vi "json Delete - string path.vi"(8 "error in (no error)":errorcluster, 10 "path":string, 11 "JSON Document in":refnum<class "JSON Document.lvclass">) -> (0 "error out":errorcluster, 1 "found?":bool, 3 "JSON Document out":refnum<class "JSON Document.lvclass">)   [LabVIEW 2015, in "JSON Document.lvclass"]
uses:
  JSON Document.lvclass
  JSON Document.lvclass/JSON Document.ctl
  rapidjson wrapper/rapidjson wrapper.lvlib
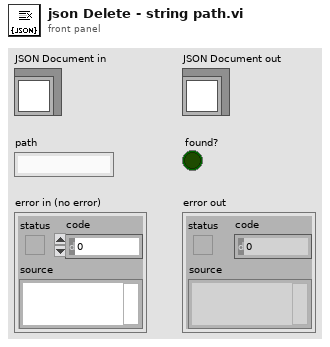
[diagram p1: front panel]
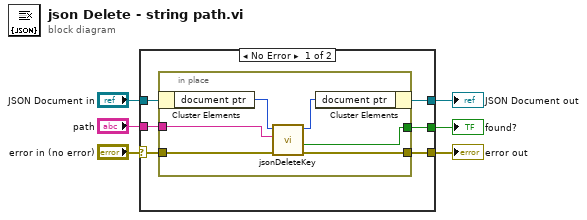
[diagram p0: block diagram]
diagram:
  n1 = case shown="No Error" "error in (no error)" {
    selector: "error in (no error)" -> [w9 w20]
    tunnel: [w8 w20] -> w5
    tunnel: [w11 w19] -> w3
    tunnel: "JSON Document in" -> [w12 w19]
    tunnel: "path" -> [w10 _]
    tunnel: [w7 _] -> w1
    frame No Error {
      n2 = in-place {
        in-place-border: w10 -> [w16]
        in-place-border: w9 -> [w15]
        in-place-border: [w14] -> w8
        in-place-border: [w13] -> w7
        n3 = in-place-cluster #1(w12) -> ("document ptr"=w18:i64)
        n4 = call "jsonDeleteKey.vi"("error in (no error)"=w15, "path"=w16, "d in"=w18) -> ("error out"=w14:errorcluster, "found?"=w13:bool, "d out"=w17:i64)  [unwired: 6 in]
        n5 = in-place-cluster #1("document ptr"=w17) -> (w11:refnum<class "JSON Document.lvclass">)
      }
    }
    frame Error {
    }
  }
  "error out" <- w5
  "JSON Document out" <- w3
  "found?" <- w1
